vi "DSF.Engine.Pool.ID.Create.vi"(7 "FIFO Debug Flags":refnum<class "Debug Flags FIFO.lvclass">, 8 "error in (no error)":errorcluster, 10 "number of IDs":u32, 11 "ID Pool type":refnum<class "DSF.Engine.Pool.ID.lvclass">) -> (0 "error out":errorcluster, 3 "ID Pool out":refnum<class "DSF.Engine.Pool.ID.lvclass">)   [LabVIEW 2017, in "Data Sharing Framework Engine.lvlib" / "DSF.Engine.Pool.ID.lvclass"]
uses:
  DSF.Engine.Pool.ID.lvclass
  C:/github/data-sharing-framework/old/dsf core/Source/Engine/Classes/Thread Pool/DSF.Engine.Pool.lvclass
  Source/Data Sharing Framework Core/Engine/Debug/Debug Flags FIFO/Debug Flags FIFO.lvclass
  DSF.Engine.Pool.lvclass/DSF.Engine.Pool.ctl
  Source/Data Sharing Framework Core/Engine/Debug/Debug Flags FIFO/Debug Flags FIFO.lvclass/Debug Flags FIFO.ctl
  DSF.Engine.Pool.Get FIFO.vi
  DSF.Engine.Pool.Get Debug Flags.vi
  Source/Data Sharing Framework Core/Engine/Debug/Debug Flags FIFO/Get Infinite Timeouts.vi
  DSF.Engine.Pool.lvclass
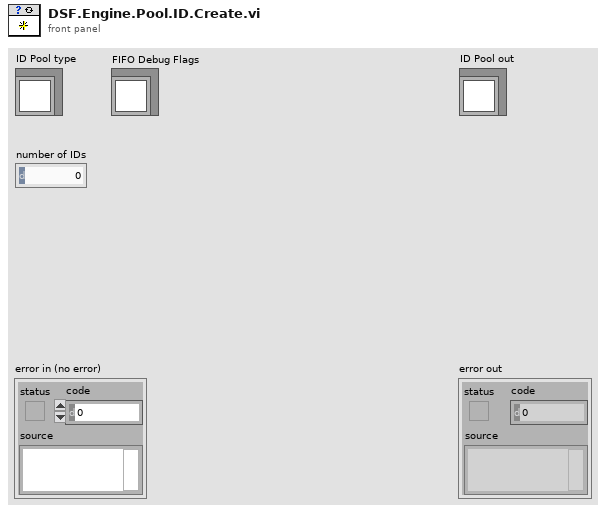
[diagram p1: front panel]
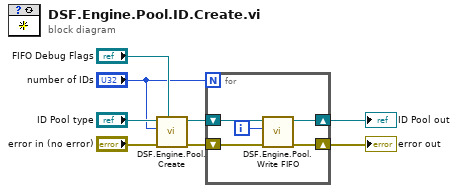
[diagram p0: block diagram]
diagram:
  n1 = call "DSF.Engine.Pool.Create.vi"("FIFO Debug Flags"="FIFO Debug Flags", "error in (no error)"="error in (no error)", "number of elements"="number of IDs", "Pool type"="ID Pool type") -> ("error out"=w3:errorcluster, "Pool"=w4:refnum<class "DSF.Engine.Pool.ID.lvclass">)  [unwired: 6 in]
  n2 = for {
    N: "number of IDs" -> [_]
    shift-right: [w11] -> w8
    shift-left: w4 -> [w13]
    shift-right: [w10] -> w7
    shift-left: w3 -> [w12]
    i -> [w9]
    n3 = call "DSF.Engine.Pool.Write FIFO.vi"("error in (no error)"=w12, "element"=w9, "Pool in"=w13) -> ("error out"=w10:errorcluster, "Pool out"=w11:refnum<class "DSF.Engine.Pool.ID.lvclass">)  [unwired: 6 in, 1 out]
  }
  "error out" <- w7
  "ID Pool out" <- w8
